vi "Start Run.vi"(8 "error in":errorcluster, 11 "class objects in":T1) -> (0 "error out":errorcluster, 1 "Notes":string, 2 "TDMS File Path":path=path "C:/Documents and Settings/pdebeule/Desktop/SpecLab RC/Integration/Test_15 Dec 2008_Pieter.tdms", 3 "class objects out":T1, 5 "Cancelled?":bool, 7 "Experiment Type":T2)   [LabVIEW 2011]
uses:
  Controls/DAQ Type.ctl
  Controls/Class Objects.ctl
  Modules/File/Configuration/Configuration.lvclass
  Modules/Hardware/Power Supply/Power Supply.lvclass
  Modules/Hardware/Mass Flow Controller/Mass Flow Controller.lvclass
  Modules/Hardware/Detector/Detector.lvclass
  Modules/Hardware/Valve Controller/Valve Controller.lvclass
  Modules/Hardware/Multimeter/Multimeter.lvclass
  Modules/File/TDMS/TDMS.lvclass
  Modules/File/Configuration/Key Data Type.ctl
panel:
  in  "Experiment Type":T2
  in  "Cancel":bool
  in  "OK":bool
  in  "Notes":string
  in  "Experiment Name":string
  in  "Operator Name":string
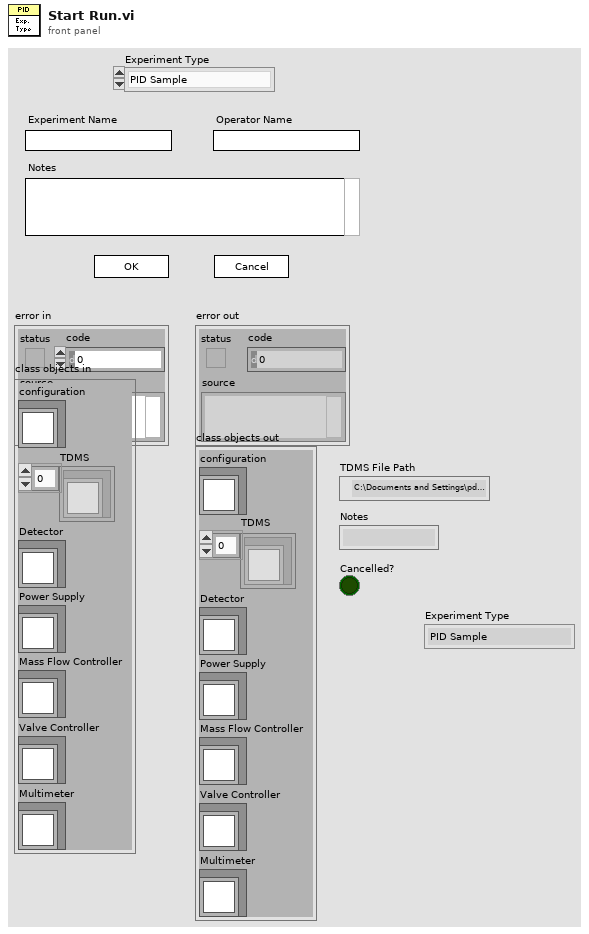
[diagram p1: front panel]
types:
  T1 = typedef "Class Objects.ctl" = cluster{"configuration":refnum<class "Configuration.lvclass">, "TDMS":refnum<class "TDMS.lvclass">[], "Detector":refnum<class "Detector.lvclass">, "Power Supply":refnum<class "Power Supply.lvclass">, "Mass Flow Controller":refnum<class "Mass Flow Controller.lvclass">, "Valve Controller":refnum<class "Valve Controller.lvclass">, "Multimeter":refnum<class "Multimeter.lvclass">}
  T2 = typedef "DAQ Type.ctl" = enum16{"PID Sample", "PID Voltage Ramp", "PID Response Time", "Multimeter Sample"}
  T3 = typedef "Configuration.lvclass/Key Data Type.ctl" = enum16{"Boolean", "U32", "I32", "Double", "String", "DAQmx Channel", "Path"}
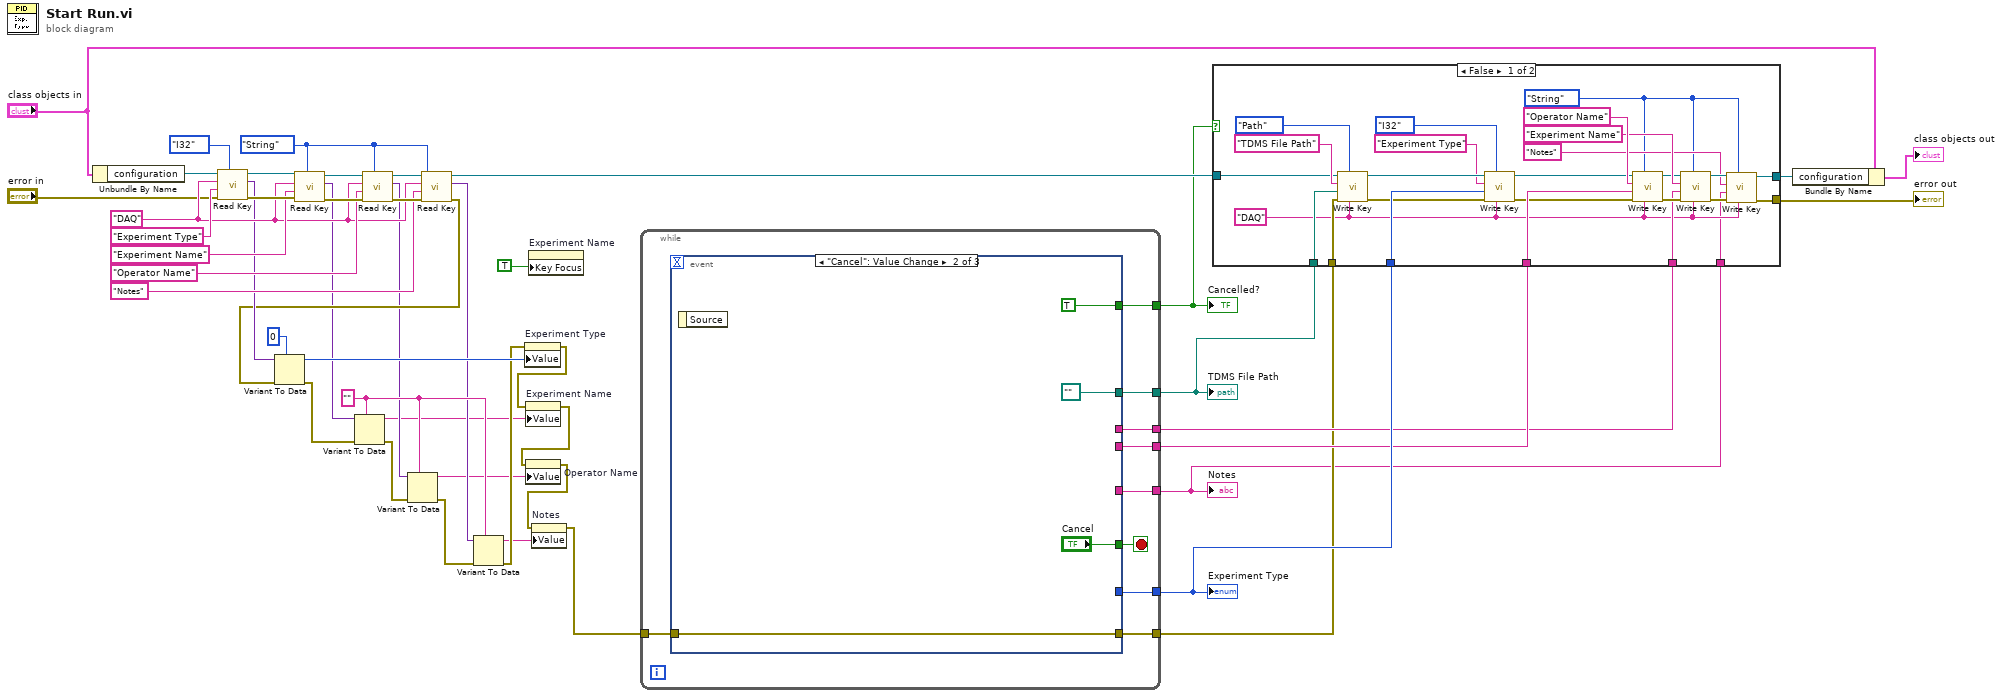
[diagram p0: block diagram]
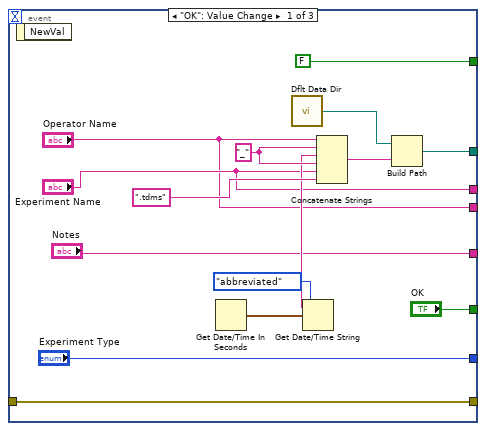
[diagram p3: hidden frame]
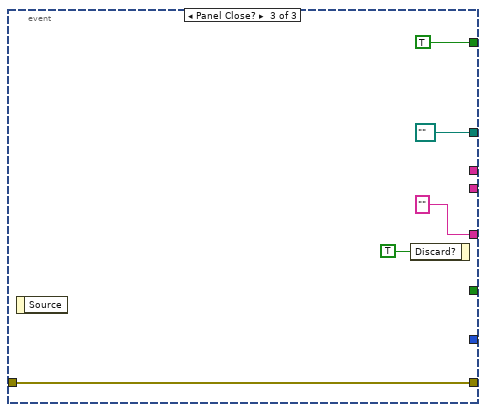
[diagram p4: hidden frame]
diagram:
  w1 = Key_Data_Type."String" ("data type")
  w20 = ""
  w26 = "DAQ" ("section")
  n1 = Unbundle By Name("class objects in") -> ("configuration"=w36:refnum<class "Configuration.lvclass">)
  n2 = call-dynamic "Read Key.vi"("data type"=Key_Data_Type."I32", "error in (no error)"="error in", "key"="Experiment Type" ("name"), "section"=w26, "Configuration.lvclass in"=w36) -> ("error out"=w31:errorcluster, "Key"=w24:variant, "Configuration.lvclass out"=w34:refnum<class "Configuration.lvclass">)  [unwired: 3 in, 1 out]
  n3 = call-dynamic "Read Key.vi"("data type"=w1, "error in (no error)"=w31, "key"="Experiment Name" ("name"), "section"=w26, "Configuration.lvclass in"=w34) -> ("error out"=w30:errorcluster, "Key"=w19:variant, "Configuration.lvclass out"=w33:refnum<class "Configuration.lvclass">)  [unwired: 3 in, 1 out]
  n4 = call-dynamic "Read Key.vi"("data type"=w1, "error in (no error)"=w30, "key"="Operator Name" ("name"), "section"=w26, "Configuration.lvclass in"=w33) -> ("error out"=w29:errorcluster, "Key"=w16:variant, "Configuration.lvclass out"=w32:refnum<class "Configuration.lvclass">)  [unwired: 3 in, 1 out]
  n5 = call-dynamic "Read Key.vi"("data type"=w1, "error in (no error)"=w29, "key"="Notes" ("name"), "section"=w26, "Configuration.lvclass in"=w32) -> ("error out"=w21:errorcluster, "Key"=w15:variant, "Configuration.lvclass out"=w4:refnum<class "Configuration.lvclass">)  [unwired: 3 in, 1 out]
  n6 = Variant To Data(error in=w21, type=0, Variant=w24) -> (data=w22:i32, error out=w18:errorcluster)
  n7 = Variant To Data(error in=w18, type=w20, Variant=w19) -> (data=w12:string, error out=w17:errorcluster)
  n8 = Variant To Data(error in=w17, type=w20, Variant=w16) -> (data=w9:string, error out=w14:errorcluster)
  n9 = Variant To Data(error in=w14, type=w20, Variant=w15) -> (data=w10:string, error out=w13:errorcluster)
  n10 = property on="Experiment Type" class="Enum (strict)"(error in=w13, "Value"=w22) -> (error out=w11:errorcluster)  [unwired: 1 in, 1 out]
  n11 = property on="Experiment Name" class="Str"(error in=w11, "Value"=w12) -> (error out=w8:errorcluster)  [unwired: 1 in, 1 out]
  n12 = property on="Operator Name" class="Str"(error in=w8, "Value"=w9) -> (error out=w7:errorcluster)  [unwired: 1 in, 1 out]
  n13 = property on="Experiment Name" class="Str"("Key Focus"=TRUE) -> ()  [unwired: 2 in, 2 out]
  n14 = property on="Notes" class="Str"(error in=w7, "Value"=w10) -> (error out=w5:errorcluster)  [unwired: 1 in, 1 out]
  n15 = while {
    tunnel: [w56] -> w42
    tunnel: [w55] -> w46
    tunnel: [w54] -> w3
    tunnel: [w53] -> w41
    tunnel: w5 -> [w52]
    tunnel: [w50] -> w45
    tunnel: [w49] -> w44
    tunnel: [w48] -> w43
    stop <- w51 stop-if-true
    n16 = event shown="[1] \"Cancel\": Value Change" {
      selector: _ -> [_ _ _]
      dyn-events: _ -> [_ _ _]
      timeout: _ -> [_ _ _]
      tunnel: w52 -> [w66 w73 w76]
      tunnel: [w66 w73 w76] -> w56
      tunnel: [w65 path "" ("appended path") path "" ("appended path")] -> w55
      tunnel: [FALSE TRUE TRUE] -> w54
      tunnel: ["Notes" _ "" ("Notes")] -> w53
      tunnel: ["OK" "Cancel" _] -> w51
      tunnel: ["Experiment Type" _ _] -> w50
      tunnel: ["Operator Name" _ _] -> w49
      tunnel: ["Experiment Name" _ _] -> w48
      event "OK": Value Change {
        w69 = "_"
        n17 = event-data() -> ()  [unwired: 1 in, 1 out]
        n18 = Get Date/Time In Seconds() -> (seconds since 1Jan1904=w67:timestamp)
        n19 = call <vilib>:"Dflt Data Dir.vi"() -> ("App:Default Data Directory"=w61:path)
        n20 = Get Date/Time String(date format (0)=enum16{"short", "long", "abbreviated"}."abbreviated", seconds (now)=w67) -> (date string=w68:string)  [unwired: 1 in, 1 out]
        n21 = Concatenate Strings("Operator Name", w69, w68, w69, "Experiment Name", ".tdms" ("string")) -> (w64:string)
        n22 = Build Path(base path=w61, name or relative path=w64) -> (appended path=w65:path)
      }
      event "Cancel": Value Change {
        n23 = event-data() -> ()  [unwired: 1 in, 1 out]
      }
      event Panel Close? {
        n24 = event-data() -> ()  [unwired: 1 in, 1 out]
        n25 = event-data("Discard?"=TRUE) -> ()  [unwired: 1 in, 1 out]
      }
    }
  }
  "TDMS File Path" <- w46
  "Cancelled?" <- w3
  "Notes" <- w41
  "Experiment Type" <- w45
  n26 = case shown="False" w3 {
    tunnel: w46 -> [w105 _]
    tunnel: w45 -> [w103 _]
    tunnel: w44 -> [w99 _]
    tunnel: w43 -> [w93 _]
    tunnel: w42 -> [w92 w107]
    tunnel: w41 -> [w87 _]
    tunnel: [w86 w107] -> w40
    tunnel: [w85 w108] -> w39
    tunnel: w4 -> [w84 w108]
    frame False {
      w81 = Key_Data_Type."String" ("data type")
      w88 = "DAQ" ("section")
      n27 = call-dynamic "Write Key.vi"("section"=w88, "data type"=Key_Data_Type."Path", "error in (no error)"=w92, "key"=w105, "name"="TDMS File Path", "Configuration.lvclass in"=w84) -> ("error out"=w97:errorcluster, "Configuration.lvclass out"=w104:refnum<class "Configuration.lvclass">)  [unwired: 4 in]
      n28 = call-dynamic "Write Key.vi"("section"=w88, "data type"=Key_Data_Type."I32", "error in (no error)"=w97, "key"=w103, "name"="Experiment Type", "Configuration.lvclass in"=w104) -> ("error out"=w98:errorcluster, "Configuration.lvclass out"=w100:refnum<class "Configuration.lvclass">)  [unwired: 4 in]
      n29 = call-dynamic "Write Key.vi"("section"=w88, "data type"=w81, "error in (no error)"=w98, "key"=w99, "name"="Operator Name", "Configuration.lvclass in"=w100) -> ("error out"=w94:errorcluster, "Configuration.lvclass out"=w95:refnum<class "Configuration.lvclass">)  [unwired: 4 in]
      n30 = call-dynamic "Write Key.vi"("section"=w88, "data type"=w81, "error in (no error)"=w94, "key"=w93, "name"="Experiment Name", "Configuration.lvclass in"=w95) -> ("error out"=w91:errorcluster, "Configuration.lvclass out"=w90:refnum<class "Configuration.lvclass">)  [unwired: 4 in]
      n31 = call-dynamic "Write Key.vi"("section"=w88, "data type"=w81, "error in (no error)"=w91, "key"=w87, "name"="Notes", "Configuration.lvclass in"=w90) -> ("error out"=w86:errorcluster, "Configuration.lvclass out"=w85:refnum<class "Configuration.lvclass">)  [unwired: 4 in]
    }
    frame True {
    }
  }
  "error out" <- w40
  n32 = Bundle By Name(cluster="class objects in", "configuration"=w39) -> (→"class objects out":T1)
